vi "题目1.vi"() -> ()   [LabVIEW 2017]
panel:
  out "元素 4":dbl
  out "元素 3":dbl
  out "元素 2":dbl
  out "元素":dbl
  out "数组":dbl[](array[numeric])
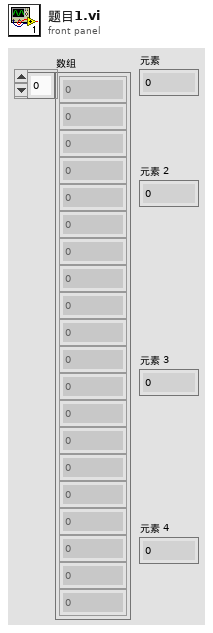
[diagram p1: front panel]
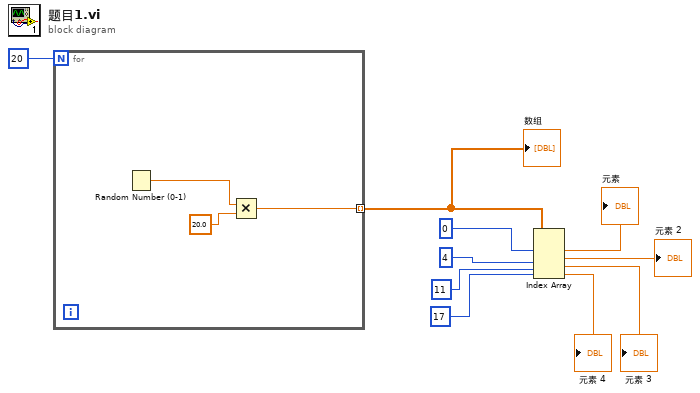
[diagram p0: block diagram]
diagram:
  n1 = for {
    N: 20 -> [_]
    tunnel: [w11] -> w9 mode=indexing
    n2 = Random Number (0-1)() -> (number: 0 to 1=w13:dbl)
    n3 = Multiply(x=w13, y=20.0) -> (x*y=w11:dbl)
  }
  "数组" <- w9
  n4 = Index Array(array=w9, index #1=0 ("索引"), index #2=4 ("索引"), index #3=11 ("索引"), index #4=17 ("索引")) -> (element #1=→"元素":dbl, element #2=→"元素 2":dbl, element #3=→"元素 3":dbl, element #4=→"元素 4":dbl)
